vi "Patch TIFF handles Gen.vi"(0 "Experimental Folder":path, 7 "No of Patches":i32) -> (4 "Cancelled":bool, 6 "Red TIFFs":path[](array[path]), 8 "Red TIFF handles":i32[](array[numeric]), 10 "Green TIFF handles":i32[](array[numeric]), 15 "Green TIFFs":path[](array[path]))   [LabVIEW 2020]
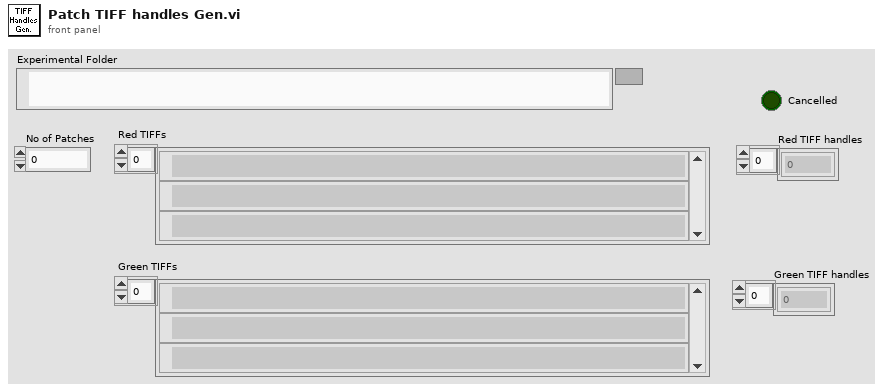
[diagram p1: front panel]
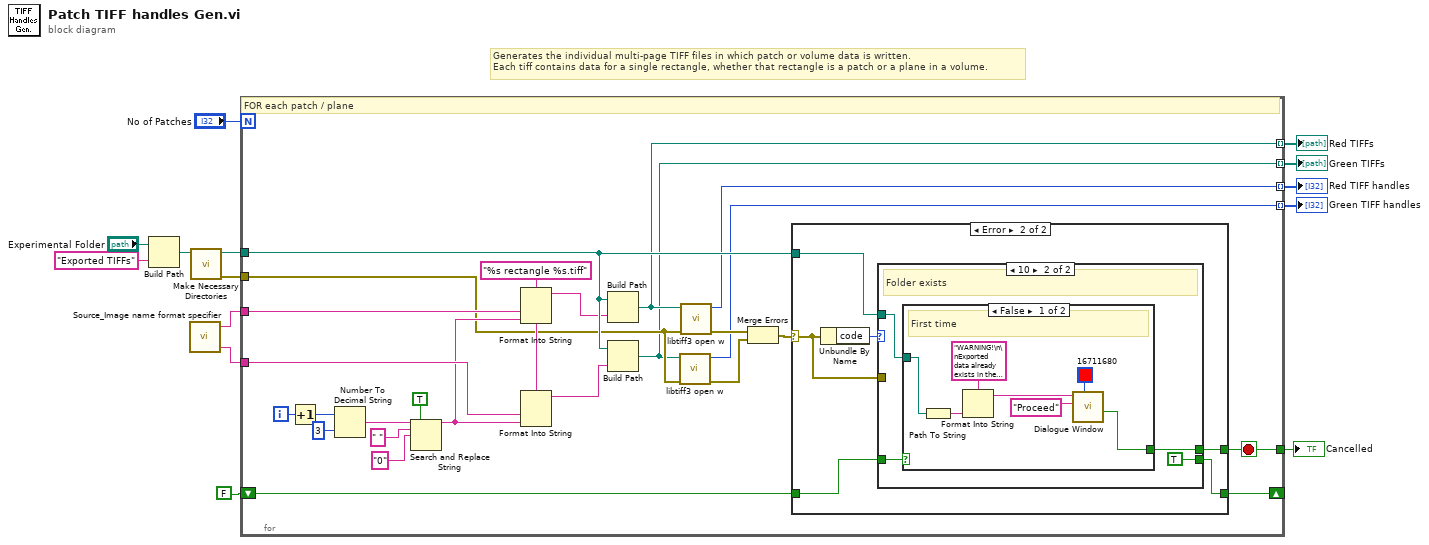
[diagram p0: block diagram]
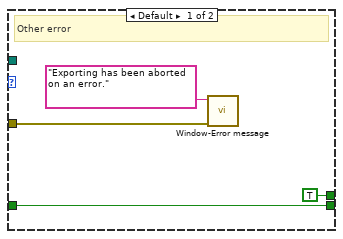
[diagram p3: hidden frame]
diagram:
  # "Generates the individual multi-page TIFF files in which patch or volume data is written.\nEach tiff contains data for a single rectangle, whether that rectangle is a patch or a plane in a volume."
  n1 = Build Path(base path="Experimental Folder", name or relative path="Exported TIFFs") -> (appended path=w8:path)
  n2 = call "Source_Image name format specifier.vi"() -> ("Red channel name"=w14:string, "Green channel name"=w13:string)  [unwired: 5 in, 1 out]
  n3 = call <userlib>:"Make Necessary Directories.vi"("Path"=w8) -> ("error out"=w6:errorcluster, "Duplicated path"=w7:path)  [unwired: 9 in]
  n4 = for {
    N: "No of Patches" -> [_]
    tunnel: w7 -> [w30]
    tunnel: w14 -> [w28]
    tunnel: w13 -> [w27]
    tunnel: [w18] -> w5 mode=indexing
    tunnel: [w17] -> w4 mode=indexing
    shift-right: [w32] -> _
    shift-left: FALSE -> [w31]
    tunnel: [w29] -> w11
    tunnel: w6 -> [w22]
    tunnel: [w16] -> w3 mode=indexing
    tunnel: [w15] -> w2 mode=indexing
    i -> [w39]
    stop <- w29 stop-if-true
    w23 = "%s rectangle %s.tiff" ("format string")
    # "FOR each patch / plane"
    n5 = Increment(x=w39) -> (x+1=w33:i32)
    n6 = Number To Decimal String(number=w33, width (-)=i16 3) -> (decimal integer string=w37:string)
    n7 = Search and Replace String(replace all?=TRUE ("replace all? (F)"), input string=w37, search string=" ", replace string="0" ("replace string (\"\")")) -> (result string=w26:string)  [unwired: 4 in, 3 out]
    n8 = Format Into String(format string=w23, w28, w26) -> (resulting string=w24:string)  [unwired: 2 in, 1 out]
    n9 = Format Into String(format string=w23, w27, w26) -> (resulting string=w25:string)  [unwired: 2 in, 1 out]
    n10 = Build Path(base path=w30, name or relative path=w24) -> (appended path=w18:path)
    n11 = Build Path(base path=w30, name or relative path=w25) -> (appended path=w17:path)
    n12 = call "libtiff3 open w.vi"("error in (no error)"=w22, "Input path"=w17) -> ("error out"=w19:errorcluster, "handle"=w15:i32)  [unwired: 8 in]
    n13 = call "libtiff3 open w.vi"("error in (no error)"=w22, "Input path"=w18) -> ("error out"=w21:errorcluster, "handle"=w16:i32)  [unwired: 8 in]
    n14 = Merge Errors(w21, w19) -> (w20:errorcluster)
    n15 = case shown="Error" w20 {
      selector: w20 -> [_ w41]
      tunnel: [w40 w45] -> w32
      tunnel: w31 -> [w40 w44]
      tunnel: w30 -> [_ w43]
      tunnel: [_ w42] -> w29
      frame No Error {
      }
      frame Error {
        n16 = Unbundle By Name(w41) -> ("code"=w46:i32)
        n17 = case shown="10" w46 {
          tunnel: [w50 TRUE] -> w45
          tunnel: w44 -> [w50 w53]
          tunnel: w43 -> [_ w52]
          tunnel: [TRUE ("Cancelled (Left button pressed)") w51] -> w42
          tunnel: w41 -> [w48 _]
          frame Default {
            # "Other error"
            n18 = call "Window-Error message.vi"("error in (no error)"=w48, "Message"="Exporting has been aborted on an error.") -> ()  [unwired: 9 in, 1 out]
          }
          frame 10 {
            # "Folder exists"
            n19 = case shown="False" w53 {
              tunnel: w52 -> [w59 _]
              tunnel: [w55 _] -> w51
              frame False {
                # "First time"
                n20 = Path To String(path=w59) -> (string=w57:string)
                n21 = Format Into String(format string="WARNING!\n\nExported data already exists in the following folder. If you proceed exported data will be overwritten.\n\n%s\n" ("Message string"), w57) -> (resulting string=w56:string)  [unwired: 2 in, 1 out]
                n22 = call "Dialogue Window.vi"("Colour"=u32 16711680, "Caption-Right button (OK)"="Proceed", "Message string"=w56) -> ("Cancelled (Left button pressed)"=w55:bool)  [unwired: 6 in, 2 out]
              }
              frame True {
                # "Acknowledged"
              }
            }
          }
        }
      }
    }
  }
  "Green TIFFs" <- w4
  "Red TIFFs" <- w5
  "Cancelled" <- w11
  "Red TIFF handles" <- w3
  "Green TIFF handles" <- w2
